vi "FormatOpcode.vi"(5 "final":bool, 8 "opcode":T1) -> (2 "opcode":string)   [LabVIEW 2014, in "Raspberry Pi Compatible Compiler for LabVIEW.lvlib" / "Websocket.lvlib"]
uses:
  Websocket.lvlib
  WebsocketFrameTypes_TD.ctl
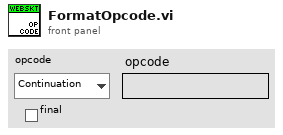
[diagram p1: front panel]
types:
  T1 = typedef "Raspberry Pi Compatible Compiler for LabVIEW.lvlib/Websocket.lvlib/WebsocketFrameTypes_TD.ctl" = enum8{"Continuation", "Text", "Binary", "Reserved 1", "Reserved 2", "Reserved 3", "Reserved 4", "Reserved 5", "Close", "Ping", "Pong", "Reserved 6", "Reserved 7", "Reserved 8", "Reserved 9", "Reserved 10"}
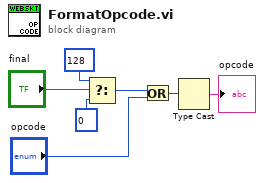
[diagram p0: block diagram]
diagram:
  n1 = Select(t=u8 128, s="final", f=u8 0 ("t")) -> (s? t:f=w4:u8)
  n2 = Or(x=w4, y="opcode") -> (x .or. y?=w2:u8)
  n3 = Type Cast(x=w2) -> (*(type *) &x=→"opcode":string)  [unwired: 1 in]
